vi "Init Group.vi"(8 "error in (no error)":errorcluster, 11 "StringGroup in":refnum<class "StringGroup.lvclass">) -> (0 "error out":errorcluster, 3 "StringGroup out":refnum<class "StringGroup.lvclass">)   [LabVIEW 2020, in "Vecto.lvlib" / "StringGroup.lvclass"]
uses:
  StringGroup.lvclass
  StringGroup.lvclass/StringGroup.ctl
  GroupAbstract/GroupAbstract.lvclass
  Group Config/Group Config.lvclass
  Ref.ctl
  C:/dev/lv20CE/relink/lv-vecto/Vecto/GroupAbstract/GroupAbstract.lvclass
  C:/dev/lv20CE/relink/lv-vecto/Vecto/StringGroup/StringGroup.lvclass
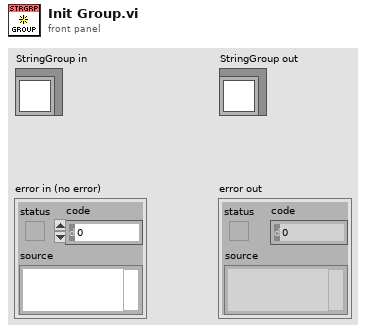
[diagram p1: front panel]
types:
  T1 = typedef "Vecto.lvlib/StringGroup.lvclass/Ref.ctl" = cluster{"Strings":string[], "Timestamp":dbl[]}
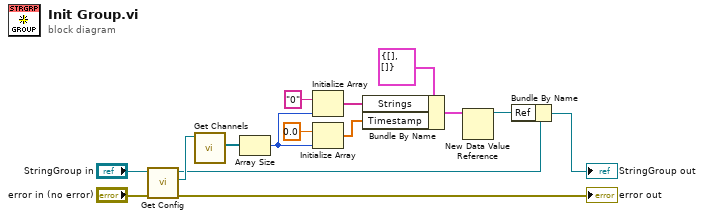
[diagram p0: block diagram]
diagram:
  n1 = call "Get Config.vi"("error in (no error)"="error in (no error)", "GroupAbstract in"="StringGroup in") -> ("error out"=→"error out":errorcluster, "Config"=w11:refnum<class "Group Config.lvclass">, "GroupAbstract out"=w3:refnum<class "StringGroup.lvclass">)  [unwired: 7 in]
  n2 = call "Get Channels.vi"("Group Config in"=w11) -> ("Channels"=w10:refnum<class "Channel Config.lvclass">[])  [unwired: 8 in, 2 out]
  n3 = Array Size(array=w10) -> (size(s)=w5:i32)
  n4 = Initialize Array("0" ("element"), w5) -> (w12:string[])
  n5 = Initialize Array(0.0 ("element"), w5) -> (w4:dbl[])
  n6 = Bundle By Name(cluster=T1 {"Strings"=[], "Timestamp"=[]} ("Ref"), "Strings"=w12, "Timestamp"=w4) -> (w14:T1)
  n7 = New Data Value Reference(data value=w14) -> (data value reference=w2:refnum<data-value>)  [unwired: 1 in, 1 out]
  n8 = Bundle By Name(cluster=w3, "Ref"=w2) -> (→"StringGroup out":refnum<class "StringGroup.lvclass">)
